vi "Corrected Range.vi"(8 "Error In":errorcluster, 10 "Channel (0)":i32, 11 "VISA resource name":refnum<visa-resource-name>) -> (0 "Error Out":errorcluster, 1 "Corrected Range":dbl[unit], 3 "dup VISA resource name":refnum<visa-resource-name>)   [LabVIEW 2012, in "MGC647C.lvlib"]
doc: "Return real range in SI units with gas correction factor included."
uses:
  <instrlib>/MGC647C/MGC647C.lvlib
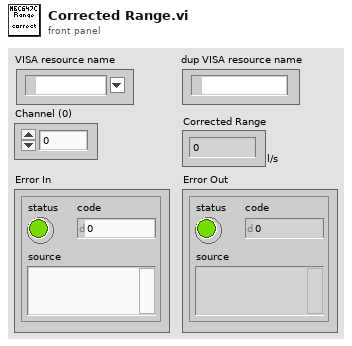
[diagram p1: front panel]
types:
  T1 = enum16{"1.000 SCCM", "2.000 SCCM", "5.000 SCCM", "10.00 SCCM", "20.00 SCCM", "50.00 SCCM", "100.0 SCCM", "200.0 SCCM", "500.0 SCCM", "1.000 SLM", "2.000 SLM", "5.000 SLM", "10.00 SLM", "20.00 SLM", "50.00 SLM", "100.0 SLM", "200.0 SLM", "400.0 SLM", "500.0 SLM", "1.000 SCMM", "1.000 SCFH", "2.000 SCFH", "5.000 SCFH", "10.00 SCFH", "20.00 SCFH", "50.00 SCFH", "100.0 SCFH", "200.0 SCFH", "500.0 SCFH", "1.000 SCFM", "2.000 SCFM", "5.000 SCFM", "10.00 SCFM", "20.00 SCFM", "50.00 SCFM", "100.0 SCFM", "200.0 SCFM", "500.0 SCFM", "30.00 SLM", "300.0 SLM"}
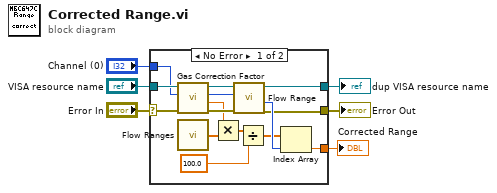
[diagram p0: block diagram]
diagram:
  n1 = case shown="No Error" "Error In" {
    selector: "Error In" -> [w16 w22]
    tunnel: "VISA resource name" -> [w15 w21]
    tunnel: [w9 w21] -> w5
    tunnel: [w8 w22] -> w4
    tunnel: "Channel (0)" -> [w14 _]
    tunnel: [w7 _] -> w1
    frame No Error {
      n2 = call <instrlib>:"Gas Correction Factor.vi"("Error In"=w16, "Channel (0)"=w14, "VISA resource name"=w15) -> ("Error Out"=w17:errorcluster, "Gas Correction Factor out"=w12:dbl, "dup VISA resource name"=w18:refnum<visa-resource-name>)  [unwired: 6 in]
      n3 = call <instrlib>:"Flow Ranges.vi"() -> ("Flow Ranges"=w20:dbl[unit][])
      n4 = Multiply(x=w12, y=w20) -> (x*y=w13:dbl[unit][])
      n5 = call <instrlib>:"Flow Range.vi"("Error In"=w17, "Channel (0)"=w14, "VISA resource name"=w18) -> ("Error Out"=w8:errorcluster, "Range out"=w19:T1, "dup VISA resource name"=w9:refnum<visa-resource-name>)  [unwired: 6 in]
      n6 = Divide(x=w13, y=100.0) -> (x/y=w11:dbl[unit][])
      n7 = Index Array(array=w11, index=w19) -> (element=w7:dbl[unit])
    }
    frame Error {
    }
  }
  "dup VISA resource name" <- w5
  "Error Out" <- w4
  "Corrected Range" <- w1
